vi "matlab.vi"   [LabVIEW 2012]
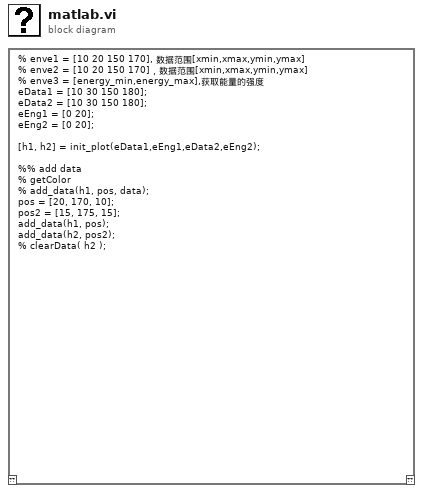
[diagram p0: block diagram]
diagram:
  n1 = script code="% enve1 = [10 20 150 170], 数据范围[xmin,xmax,ymin,ymax]\n% enve2 = [10 20 150 170]，数据范围[xmin,xmax,ymin,ymax]\n% enve3 = [energy_min,energy_max],获取能量的强度\neData1 = [10 30 150 180];\neData2 = [10 30 150 180];\neEng1 = [0 20];\neEng2 = [0 20];\n\n[h1, h2] = init_plot(eData1,eEng1,eData2,eEng2);\n\n%% add data\n% getColor\n% add_data(h1, pos, data);\npos = [20, 170, 10];\npos2 = [15, 175, 15];\nadd_data(h1, pos);\nadd_data(h2, pos2);\n% clearData( h2 );"() -> ()  [unwired: 1 in, 1 out]
